vi "Configure Resolution and Video Bandwidth.vi"(8 "error in (no error)":errorcluster, 9 "VBW [Hz]":dbl, 10 "RBW [Hz]":dbl, 11 "SA-FSW in":refnum<class "SA-FSW.lvclass">) -> (0 "error out":errorcluster, 3 "SA-FSW out":refnum<class "SA-FSW.lvclass">)   [LabVIEW 2020, in "SA-FSW.lvclass"]
uses:
  SA-FSW.lvclass
  C:/Sandbox/Git_Sandbox/WiSpry Test Framework source code (LV20)/WiSpry Test Framework/Instruments/Instrument.lvclass
  C:/Sandbox/Git_Sandbox/WiSpry Test Framework source code (LV20)/WiSpry Test Framework/Instruments/Spectrum Analyzer/Spectrum Analyzer.lvclass
  Instrument.lvclass/Instrument.ctl
  Spectrum Analyzer.lvclass/Spectrum Analyzer.ctl
  Instrument.lvclass
  Spectrum Analyzer.lvclass
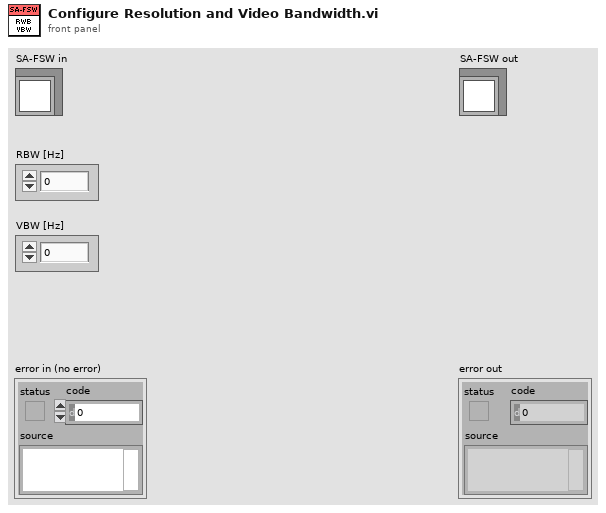
[diagram p1: front panel]
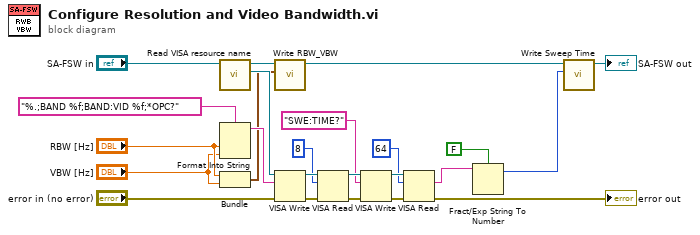
[diagram p0: block diagram]
diagram:
  n1 = call "Read VISA resource name.vi"("Instrument in"="SA-FSW in") -> ("VISA resource name"=w22:refnum<visa-resource-name>, "Instrument out"=w16:refnum<class "SA-FSW.lvclass">)  [unwired: 9 in]
  n2 = Format Into String(format string="%.;BAND %f;BAND:VID %f;*OPC?" ("initial string"), "RBW [Hz]", "VBW [Hz]") -> (resulting string=w21:string)  [unwired: 2 in, 1 out]
  n3 = Bundle("RBW [Hz]"="RBW [Hz]", "VBW [Hz]"="VBW [Hz]") -> (w13:cluster{"RBW [Hz]":dbl, "VBW [Hz]":dbl})  [unwired: 1 in]
  n4 = call "Write RBW_VBW.vi"("RBW/VBW"=w13, "Spectrum Analyzer in"=w16) -> ("Spectrum Analyzer out"=w12:refnum<class "SA-FSW.lvclass">)  [unwired: 9 in]
  n5 = VISA Write(VISA resource name=w22, write buffer=w21, error in (no error)="error in (no error)") -> (VISA resource name out=w18:refnum<visa-resource-name>, error out=w19:errorcluster)  [unwired: 1 out]
  n6 = VISA Read(VISA resource name=w18, byte count=u32 8, error in (no error)=w19) -> (VISA resource name out=w10:refnum<visa-resource-name>, error out=w11:errorcluster)  [unwired: 2 out]
  n7 = VISA Write(VISA resource name=w10, write buffer="SWE:TIME?", error in (no error)=w11) -> (VISA resource name out=w7:refnum<visa-resource-name>, error out=w8:errorcluster)  [unwired: 1 out]
  n8 = VISA Read(VISA resource name=w7, byte count=u32 64, error in (no error)=w8) -> (read buffer=w4:string, error out=→"error out":errorcluster)  [unwired: 2 out]
  n9 = Fract/Exp String To Number(use system decimal point (T)=FALSE, string=w4) -> (offset past number=w1:i32)  [unwired: 2 in, 1 out]
  n10 = call "Write Sweep Time.vi"("Sweep Time"=w1, "Spectrum Analyzer in"=w12) -> ("Spectrum Analyzer out"=→"SA-FSW out":refnum<class "SA-FSW.lvclass">)  [unwired: 9 in]
